vi "Extract Qualified Paths.vi"(0 "Scalar SG SC2250 Path Group in":refnum<class "SG SC2250 Path Group.lvclass">, 5 "Paths in":refnum<class "Path.lvclass">[](array[class]), 11 "error in (no error)":errorcluster) -> (4 "Scalar SG SC2250 Path Group out":refnum<class "SG SC2250 Path Group.lvclass">, 6 "Qualified Path Count out":i32, 15 "error out":errorcluster)   [LabVIEW 2023, in "RFFixtureCharact.RFPM.lvlib" / "SG SC2250 Path Group.lvclass"]
uses:
  SG SC2250 Path Group.lvclass
  Common/Base Classes/Path/Path.lvclass
  Paths/SG SC2250 Path/SG SC2250 Path.lvclass
  C:/srd-semi-rfcal-software/AuxTools/STSRFFixtureCharactUtility/Source/Code Modules/Common/Base Classes/Path/Path.lvclass
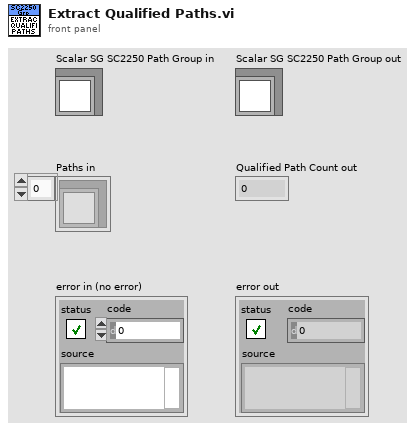
[diagram p1: front panel]
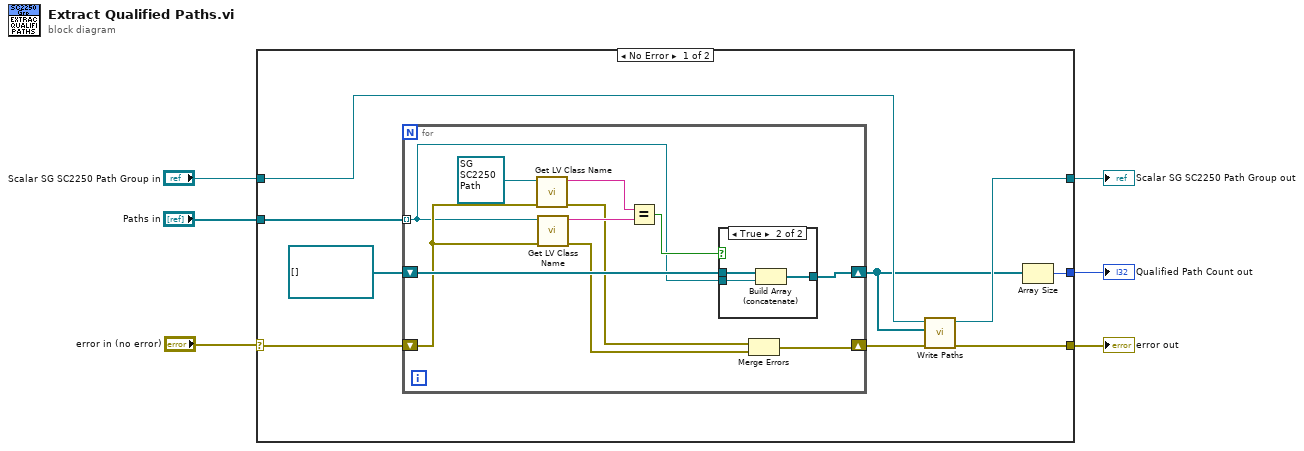
[diagram p0: block diagram]
diagram:
  n1 = case shown="No Error" "error in (no error)" {
    selector: "error in (no error)" -> [w13 w32]
    tunnel: [w10 w32] -> w5
    tunnel: [w9 w31] -> w3
    tunnel: "Paths in" -> [w14 _]
    tunnel: "Scalar SG SC2250 Path Group in" -> [w15 w31]
    tunnel: [w7 _] -> w1
    frame No Error {
      n2 = for {
        shift-right: [w23] -> w8
        shift-left: refnum<class "SG SC2250 Path.lvclass">[] [] -> [w21]
        tunnel: w14 -> [w19] mode=indexing
        shift-right: [w18] -> w11
        shift-left: w13 -> [w20]
        n3 = call <vilib>:"Get LV Class Name.vi"("error in (no error)"=w20, "object"=refnum<class "SG SC2250 Path.lvclass"> refnum ("STSScalarFixtureCharacterization.lvlib:Scalar SG SC2250 Path.lvclass")) -> ("error out"=w17:errorcluster, "class name"=w26:string)  [unwired: 8 in]
        n4 = call <vilib>:"Get LV Class Name.vi"("error in (no error)"=w20, "object"=w19) -> ("error out"=w16:errorcluster, "class name"=w25:string)  [unwired: 8 in]
        n5 = Equal?(x=w26, y=w25) -> (x = y?=w24:bool)
        n6 = case shown="True" w24 {
          tunnel: w21 -> [w27 w29]
          tunnel: [w27 w30] -> w23
          tunnel: w19 -> [_ w28]
          frame False {
          }
          frame True {
            n7 = Build Array (concatenate)(w29, w28) -> (w30:refnum<class "Path.lvclass">[])
          }
        }
        n8 = Merge Errors(w17, w16) -> (w18:errorcluster)
      }
      n9 = call-dynamic "Write Paths.vi"("error in (no error)"=w11, "Paths"=w8, "Cable Path Group in"=w15) -> ("error out"=w10:errorcluster, "Cable Path Group out"=w9:refnum<class "SG SC2250 Path Group.lvclass">)  [unwired: 7 in]
      n10 = Array Size(array=w8) -> (size(s)=w7:i32)
    }
    frame Error {
    }
  }
  "error out" <- w5
  "Scalar SG SC2250 Path Group out" <- w3
  "Qualified Path Count out" <- w1
